vi "Report Error.vi"(8 "error in (no error)":errorcluster, 9 "Message (None)":string, 11 "Module in":refnum<class "Module.lvclass">) -> (0 "error out":errorcluster, 3 "Module out":refnum<class "Module.lvclass">)   [LabVIEW 2020, in "Volatus.lvlib" / "Module.lvclass"]
uses:
  Module.lvclass
  Module.lvclass/Module.ctl
  VolatusAPI/VolatusAPI.lvclass
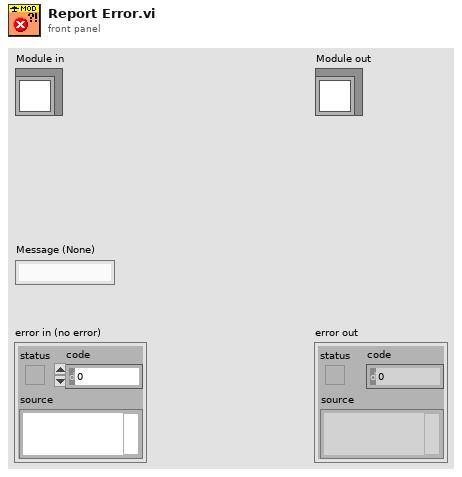
[diagram p1: front panel]
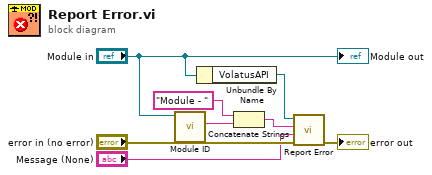
[diagram p0: block diagram]
diagram:
  n1 = call-dynamic "Module ID.vi"("Module in"="Module in") -> ("Module ID"=w3:string)  [unwired: 10 in]
  n2 = Unbundle By Name("Module in") -> ("VolatusAPI"=w8:refnum<class "VolatusAPI.lvclass">)
  n3 = Concatenate Strings("Module - ", w3) -> (w1:string)
  n4 = call "Report Error.vi"("error in (no error)"="error in (no error)", "Message"="Message (None)", "Context"=w1, "VolatusAPI in"=w8) -> ("error out"=→"error out":errorcluster)  [unwired: 6 in, 1 out]
  "Module out" <- "Module in"
